vi "read_temps(SubVI).vi"(11 "VISA Refnum in":refnum<visa-resource-name>) -> (3 "Array":dbl[](array[numeric]))   [LabVIEW 2012]
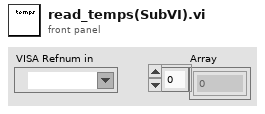
[diagram p1: front panel]
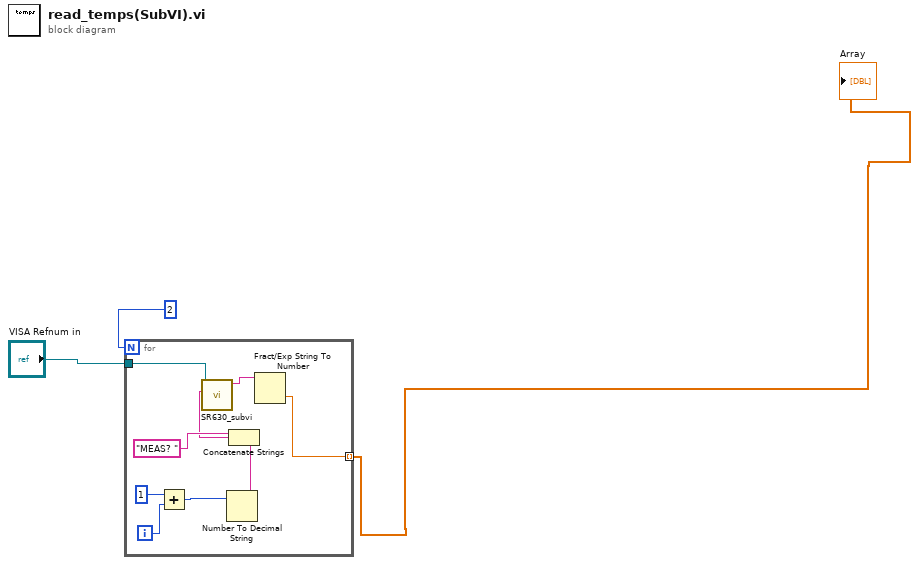
[diagram p0: block diagram]
diagram:
  n1 = for {
    N: 2 ("dimension size") -> [_]
    tunnel: "VISA Refnum in" -> [w12]
    tunnel: [w10] -> w3 mode=indexing
    i -> [w9]
    n2 = Add(x=1, y=w9) -> (x+y=w7:i32)
    n3 = Number To Decimal String(number=w7) -> (decimal integer string=w6:string)  [unwired: 1 in]
    n4 = Concatenate Strings("MEAS? " ("Write Buffer"), w6) -> (w4:string)
    n5 = call "SR630_subvi.vi"("Write Buffer"=w4, "VISA Refnum in"=w12) -> ("read buffer"=w11:string)  [unwired: 9 in]
    n6 = Fract/Exp String To Number(string=w11) -> (number=w10:dbl)  [unwired: 3 in, 1 out]
  }
  "Array" <- w3
